vi "Read BMS Data.vi"(8 "error in (no error)":errorcluster, 11 "Orion_BMS in":refnum<class "Orion_BMS.lvclass">) -> (0 "error out":errorcluster, 2 "BMS Data":T1, 3 "Orion_BMS out":refnum<class "Orion_BMS.lvclass">)   [LabVIEW 2017, in "Orion_BMS.lvclass"]
uses:
  Orion_BMS.lvclass
  TypeDef_BMSData.ctl
  TypeDef_BMS_Status.ctl
  Orion_BMS.lvclass/Orion_BMS.ctl
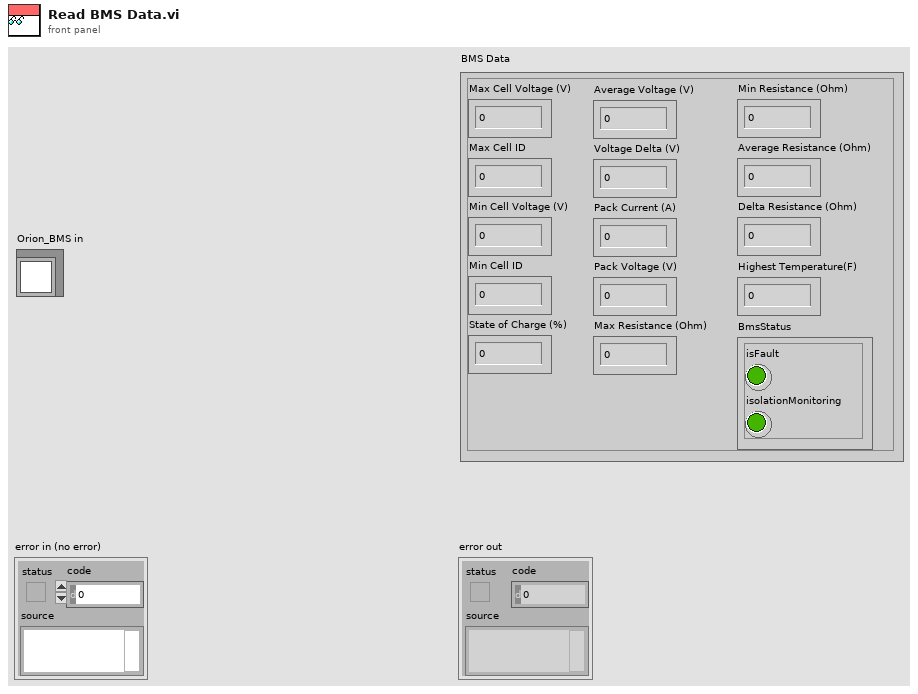
[diagram p1: front panel]
types:
  T1 = typedef "TypeDef_BMSData.ctl" = cluster{"Max Cell Voltage (V)":dbl, "Max Cell ID":dbl, "Min Cell Voltage (V)":dbl, "Min Cell ID":dbl, "State of Charge (%)":dbl, "Average Voltage (V)":dbl, "Voltage Delta (V)":dbl, "Pack Current (A)":dbl, "Pack Voltage (V)":dbl, "Max Resistance (Ohm)":dbl, "Min Resistance (Ohm)":dbl, "Average Resistance (Ohm)":dbl, "Delta Resistance (Ohm)":dbl, "Highest Temperature(F)":dbl, "BmsStatus":T2}
  T2 = typedef "TypeDef_BMS_Status.ctl" = cluster{"isFault":bool, "isolationMonitoring":bool}
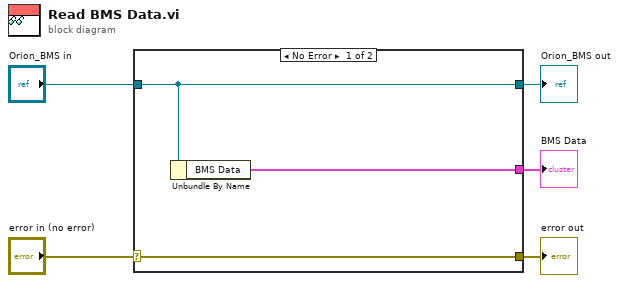
[diagram p0: block diagram]
diagram:
  n1 = case shown="No Error" "error in (no error)" {
    selector: "error in (no error)" -> [w8 w9]
    tunnel: [w8 w9] -> w4
    tunnel: [w7 w10] -> w2
    tunnel: "Orion_BMS in" -> [w7 w10]
    tunnel: [w6 _] -> w1
    frame No Error {
      n2 = Unbundle By Name(w7) -> ("BMS Data"=w6:T1)
    }
    frame Error {
    }
  }
  "error out" <- w4
  "Orion_BMS out" <- w2
  "BMS Data" <- w1
